vi "Send Batch Messages To Specific Target.vi"(8 "error in (no error)":errorcluster, 9 "Mail Strategy In":refnum<class "Mail Strategy.lvclass">, 10 "Messages In":refnum<class "Message.lvclass">[](array[class]), 11 "Messenger in":refnum<class "Simple Tree Queue Messenger.lvclass">) -> (0 "error out":errorcluster, 3 "Messenger out":refnum<class "Simple Tree Queue Messenger.lvclass">)   [LabVIEW 2019, in "Simple Tree Queue Messenger.lvclass"]
uses:
  Simple Tree Queue Messenger.lvclass
  C:/Users/iio/Desktop/NTHU Brain Center/General Library/Ancestor Class/Messenger/Messenger Composite/Messenger Composite.lvclass
  Ancestor Class/Message/Message.lvclass
  Ancestor Class/Messenger/Mail Strategy/Mail Strategy.lvclass
  Simple Tree Queue Mailman/Simple Tree Queue Mailman.lvclass
  C:/Users/iio/Desktop/NTHU Brain Center/General Library/Ancestor Class/Messenger/Mail Strategy/Mail Strategy.lvclass
  Ancestor Class/Messenger/Messenger Composite/Messenger Composite.lvclass/Messenger Composite.ctl
  Simple Tree Queue Mailman/Simple Tree Queue Mailman.lvclass/Simple Tree Queue Mailman.ctl
  Simple Tree Queue Messenger.lvclass/Simple Tree Queue Messenger.ctl
  Simple Tree Queue Mailman/Public Data/Write Address Recursive Access.vi
  Ancestor Class/Messenger/Messenger Composite/Public Data/Read Nodes.vi
  Ancestor Class/Messenger/Messenger/Messenger.lvclass
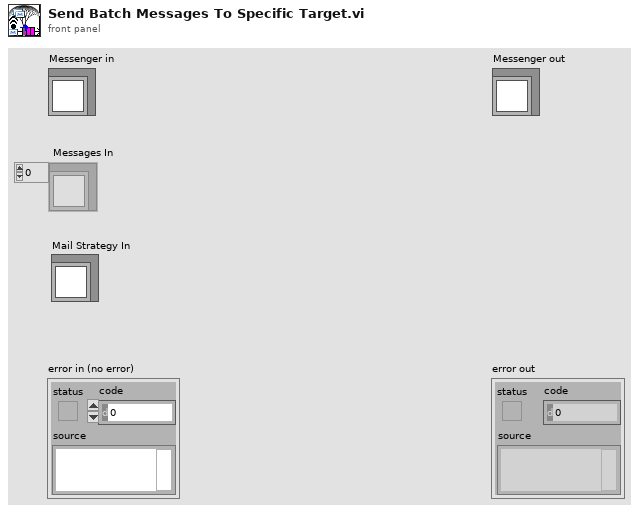
[diagram p1: front panel]
types:
  T1 = typedef "Message Queue.ctl" = refnum<queue>
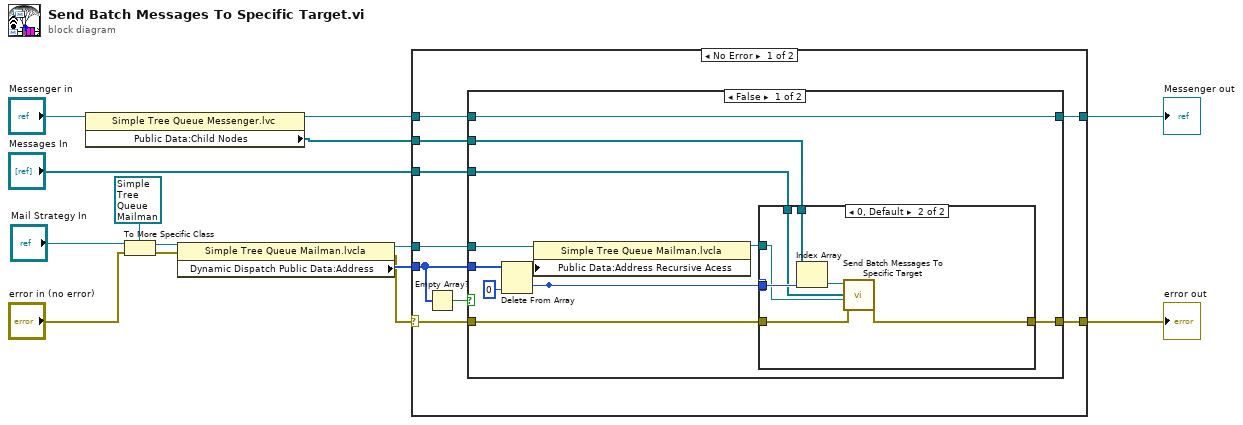
[diagram p0: block diagram]
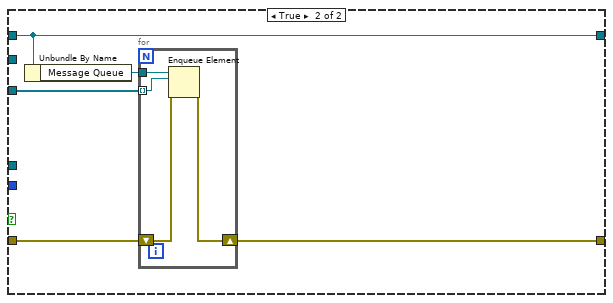
[diagram p3: hidden frame]
diagram:
  n1 = property class="Simple Tree Queue Messenger.lvc"(reference="Messenger in") -> (reference out=w3:refnum<class "Simple Tree Queue Messenger.lvclass">, "Public Data:Child Nodes"=w2:refnum<class "Messenger.lvclass">[])  [unwired: 1 in, 1 out]
  n2 = To More Specific Class(target class=refnum<class "Simple Tree Queue Mailman.lvclass"> refnum ("Array Location Mailman.lvclass"), reference="Mail Strategy In", error in="error in (no error)") -> (specific class reference=w8:refnum<class "Simple Tree Queue Mailman.lvclass">, error out=w9:errorcluster)
  n3 = property class="Simple Tree Queue Mailman.lvcla"(reference=w8, error in=w9) -> (reference out=w1:refnum<class "Simple Tree Queue Mailman.lvclass">, error out=w6:errorcluster, "Dynamic Dispatch Public Data:Address"=w7:i32[])
  n4 = case shown="No Error" w6 {
    selector: w6 -> [w18 w52]
    tunnel: w3 -> [w22 w53]
    tunnel: [w20 w53] -> w14
    tunnel: [w17 w52] -> w13
    tunnel: w7 -> [w19 _]
    tunnel: "Messages In" -> [w21 _]
    tunnel: w2 -> [w16 _]
    tunnel: w1 -> [w15 _]
    frame No Error {
      n5 = Empty Array?(array=w19) -> (empty?=w23:bool)
      n6 = case shown="False" w23 {
        tunnel: w22 -> [w34 w47]
        tunnel: w21 -> [w29 w45]
        tunnel: [w34 w47] -> w20
        tunnel: w19 -> [w33 _]
        tunnel: w18 -> [w31 w44]
        tunnel: [w30 w43] -> w17
        tunnel: w16 -> [w28 _]
        tunnel: w15 -> [w27 _]
        frame False {
          n7 = Delete From Array(array=w33, index=0) -> (deleted portion=w24:i32, array with subset deleted=w26:i32[])  [unwired: 1 in]
          n8 = property class="Simple Tree Queue Mailman.lvcla"(reference=w27, "Public Data:Address Recursive Acess"=w26) -> (reference out=w25:refnum<class "Simple Tree Queue Mailman.lvclass">)  [unwired: 1 in, 1 out]
          n9 = case shown="0, Default" w24 {
            tunnel: w24 -> [_ w42]
            tunnel: w31 -> [w35 w40]
            tunnel: [w35 w39] -> w30
            tunnel: w29 -> [_ w38]
            tunnel: w28 -> [_ w37]
            tunnel: w25 -> [_ w36]
            frame -2147483648..-1 {
            }
            frame 0, Default {
              n10 = Index Array(array=w37, index=w42) -> (element=w41:refnum<class "Messenger.lvclass">)
              n11 = call-dynamic "Send Batch Messages To Specific Target.vi"("error in (no error)"=w40, "Mail Strategy In"=w36, "Messages In"=w38, "Messenger in"=w41) -> ("error out"=w39:errorcluster)  [unwired: 6 in, 1 out]
            }
          }
        }
        frame True {
          n12 = Unbundle By Name(w47) -> ("Message Queue"=w46:T1)
          n13 = for {
            tunnel: w46 -> [w51]
            tunnel: w45 -> [w50] mode=indexing
            shift-right: [w48] -> w43
            shift-left: w44 -> [w49]
            n14 = Enqueue Element(queue=w51, element=w50, error in (no error)=w49) -> (error out=w48:errorcluster)  [unwired: 1 in, 2 out]
          }
        }
      }
    }
    frame Error {
    }
  }
  "error out" <- w13
  "Messenger out" <- w14
